vi "is_alfa.vi"(1 "char":u8 format="%02x") -> (0 "isAlfa":bool)   [LabVIEW 2011]
panel:
  out "string":string
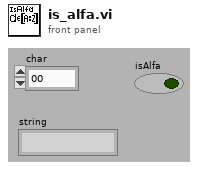
[diagram p1: front panel]
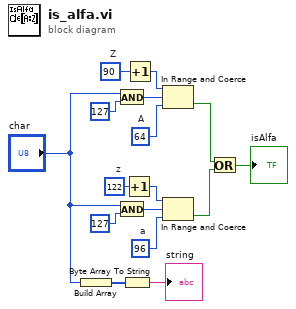
[diagram p0: block diagram]
diagram:
  w1 = u8 122  # z
  w12 = u8 96  # a
  w3 = u8 90  # Z
  w16 = u8 64  # A
  n1 = Build Array("char") -> (w7:u8[])
  n2 = And(x="char", y=u8 127) -> (x .and. y?=w5:u8)
  n3 = And(x="char", y=u8 127) -> (x .and. y?=w13:u8)
  n4 = Byte Array To String(unsigned byte array=w7) -> (string=→"string":string)
  n5 = Increment(x=w1) -> (x+1=w2:u8)
  n6 = Increment(x=w3) -> (x+1=w4:u8)
  n7 = In Range and Coerce(upper limit=w4, x=w5, lower limit=w16) -> (In Range?=w11:bool)  [unwired: 1 out]
  n8 = In Range and Coerce(upper limit=w2, x=w13, lower limit=w12) -> (In Range?=w10:bool)  [unwired: 1 out]
  n9 = Or(x=w11, y=w10) -> (x .or. y?=→"isAlfa":bool)
